vi "GetContent.vi"(8 "Error In":errorcluster, 11 "reference in":refnum<class "ItalicDecorator.lvclass">) -> (0 "Error Out":errorcluster, 2 "Content":string, 3 "reference out":refnum<class "ItalicDecorator.lvclass">)   [LabVIEW 2024, in "ItalicDecorator.lvclass"]
uses:
  ItalicDecorator.lvclass
  ItalicDecorator.lvclass/ItalicDecorator.ctl
  AbstractText/AbstractText.lvclass
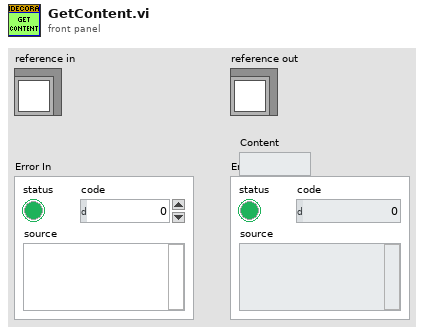
[diagram p1: front panel]
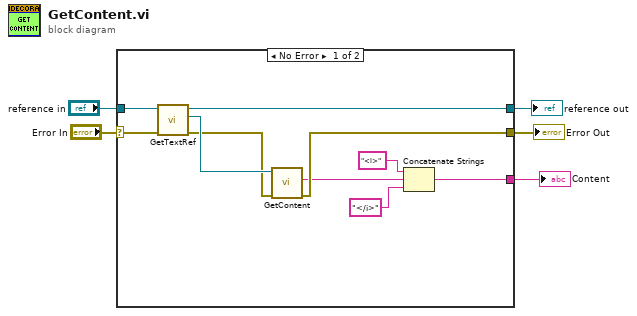
[diagram p0: block diagram]
diagram:
  n1 = case shown="No Error" "Error In" {
    selector: "Error In" -> [w15 w17]
    tunnel: [w10 w17] -> w4
    tunnel: [w13 w16] -> w2
    tunnel: "reference in" -> [w14 w16]
    tunnel: [w6 _] -> w1
    frame No Error {
      n2 = call-dynamic "GetTextRef.vi"("Error In"=w15, "reference in"=w14) -> ("Error Out"=w11:errorcluster, "TextRef"=w12:refnum<class "AbstractText.lvclass">, "reference out"=w13:refnum<class "ItalicDecorator.lvclass">)  [unwired: 7 in]
      n3 = call-dynamic "GetContent.vi"("Error In"=w11, "reference in"=w12) -> ("Error Out"=w10:errorcluster, "Content"=w9:string)  [unwired: 7 in, 1 out]
      n4 = Concatenate Strings("<i>" ("string"), w9, "</i>" ("string")) -> (w6:string)
    }
    frame Error {
    }
  }
  "Error Out" <- w4
  "reference out" <- w2
  "Content" <- w1
